vi "Configure Trigger Coupling.vi"(8 "error in (no error)":errorcluster, 9 "Trigger Coupling (4: DC)":u16(ring)=4 items=["AC1M", "DC1M", "DC50", "Ground", "DC", "AC", "LFREJ", "HFREJ", "HF"], 10 "Trigger Source (0: Channel 1)":u16(ring) items=["Channel 1", "Channel 2", "Channel 3", "Channel 4", "Ext", "Ext10"], 11 "VISA resource name":refnum<visa-resource-name>) -> (0 "error out":errorcluster, 3 "VISA resource name out":refnum<visa-resource-name>)   [LabVIEW 2015, in "LeCroy Wave Series.lvlib"]
doc: "Sets the coupling mode of the specified trigger source."
uses:
  <instrlib>/LeCroy Wave Series/LeCroy Wave Series.lvlib
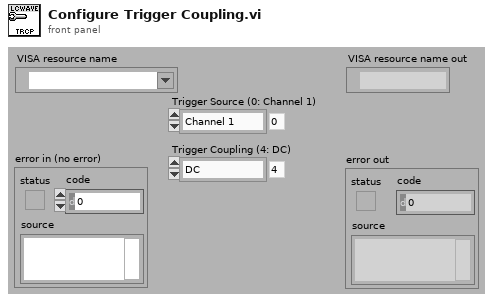
[diagram p1: front panel]
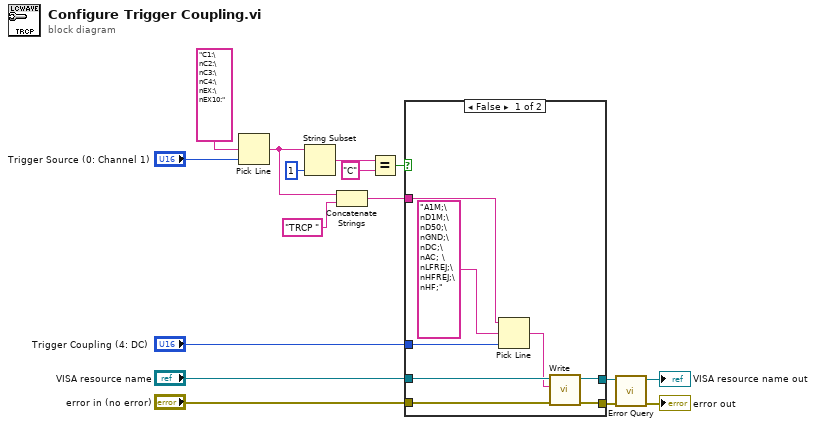
[diagram p0: block diagram]
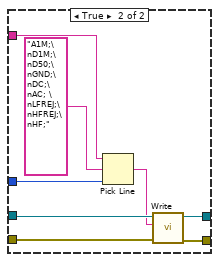
[diagram p2: hidden frame]
diagram:
  n1 = Pick Line(multi-line string="C1:\nC2:\nC3:\nC4:\nEX:\nEX10:", line index="Trigger Source (0: Channel 1)") -> (output string=w3:string)  [unwired: 1 in]
  n2 = String Subset(string=w3, length (rest)=1 ("length (rest)")) -> (substring=w13:string)  [unwired: 1 in]
  n3 = Concatenate Strings(w3, "TRCP ") -> (w1:string)
  n4 = Equal?(x=w13, y="C") -> (x = y?=w11:bool)
  n5 = case shown="False" w11 {
    tunnel: [w22 w32] -> w7
    tunnel: [w21 w31] -> w4
    tunnel: w1 -> [w18 w28]
    tunnel: "VISA resource name" -> [w24 w30]
    tunnel: "error in (no error)" -> [w23 w29]
    tunnel: "Trigger Coupling (4: DC)" -> [w20 w25]
    frame False {
      n6 = Pick Line(string ("")=w18, multi-line string="A1M;\nD1M;\nD50;\nGND;\nDC;\nAC; \nLFREJ;\nHFREJ;\nHF;", line index=w20) -> (output string=w19:string)
      n7 = call <instrlib>:"Write.vi"("error in (no error)"=w23, "Write Buffer"=w19, "VISA resource name"=w24) -> ("error out"=w21:errorcluster, "VISA resource name out"=w22:refnum<visa-resource-name>)  [unwired: 6 in, 1 out]
    }
    frame True {
      n8 = Pick Line(string ("")=w28, multi-line string="A1M;\nD1M;\nD50;\nGND;\nDC;\nAC; \nLFREJ;\nHFREJ;\nHF;", line index=w25) -> (output string=w27:string)
      n9 = call <instrlib>:"Write.vi"("error in (no error)"=w29, "Write Buffer"=w27, "VISA resource name"=w30) -> ("error out"=w31:errorcluster, "VISA resource name out"=w32:refnum<visa-resource-name>)  [unwired: 6 in, 1 out]
    }
  }
  n10 = call <instrlib>:"Error Query.vi"("error in (no error)"=w4, "VISA resource name"=w7) -> ("error out"=→"error out":errorcluster, "VISA resource name out"=→"VISA resource name out":refnum<visa-resource-name>)  [unwired: 6 in, 2 out]
